vi "Update Default Template from Metadata.vi"(8 "error in":errorcluster, 9 "project refnum":refnum<vi>, 10 "measurement_signature":T2, 11 "gRPCid in":T1) -> (0 "error out":errorcluster, 1 "default value":variant, 2 "copy template path":path, 3 "gRPCid out":T1)   [LabVIEW 2021, in "MeasurementClient Editor.lvlib"]
uses:
  MeasurementClient Editor.lvlib
  <vilib>/gRPC/Generated APIs/ni/measurementlink/measurement/v2/Measurement Service Client V2/RPC Messages/ni_measurementlink_measurement_v2_MeasurementSignature.ctl
  <vilib>/gRPC/Generated APIs/ni/measurementlink/measurement/v2/Measurement Service Client V2/RPC Messages/ni_measurementlink_measurement_v2_ConfigurationParameter.ctl
  <vilib>/gRPC/Generated APIs/ni/measurementlink/measurement/v2/Measurement Service Client V2/RPC Messages/google_protobuf_Field_Kind.ctl
  <vilib>/gRPC/Generated APIs/ni/measurementlink/measurement/v2/Measurement Service Client V2/RPC Messages/ni_measurementlink_measurement_v2_ConfigurationParameter_AnnotationsEntry.ctl
  <vilib>/gRPC/Generated APIs/ni/measurementlink/measurement/v2/Measurement Service Client V2/RPC Messages/google_protobuf_Any.ctl
  <vilib>/gRPC/Generated APIs/ni/measurementlink/measurement/v2/Measurement Service Client V2/RPC Messages/ni_measurementlink_measurement_v2_Output.ctl
  <vilib>/gRPC/Generated APIs/ni/measurementlink/measurement/v2/Measurement Service Client V2/RPC Messages/ni_measurementlink_measurement_v2_Output_AnnotationsEntry.ctl
  <vilib>/gRPC/LabVIEW gRPC Library/Shared/grpcId.ctl
  <vilib>/Utility/traverseref.llb/TRef TravTarget.ctl
  <vilib>/gRPC/LabVIEW gRPC Library/grpc-lvsupport-release.lvlib
  <vilib>/Utility/traverseref.llb/VI Scripting - Traverse.lvlib
  <vilib>/gRPC/Generated APIs/ni/measurementlink/measurement/v2/Measurement Service Client V2/Measurement Service Client V2.lvlib
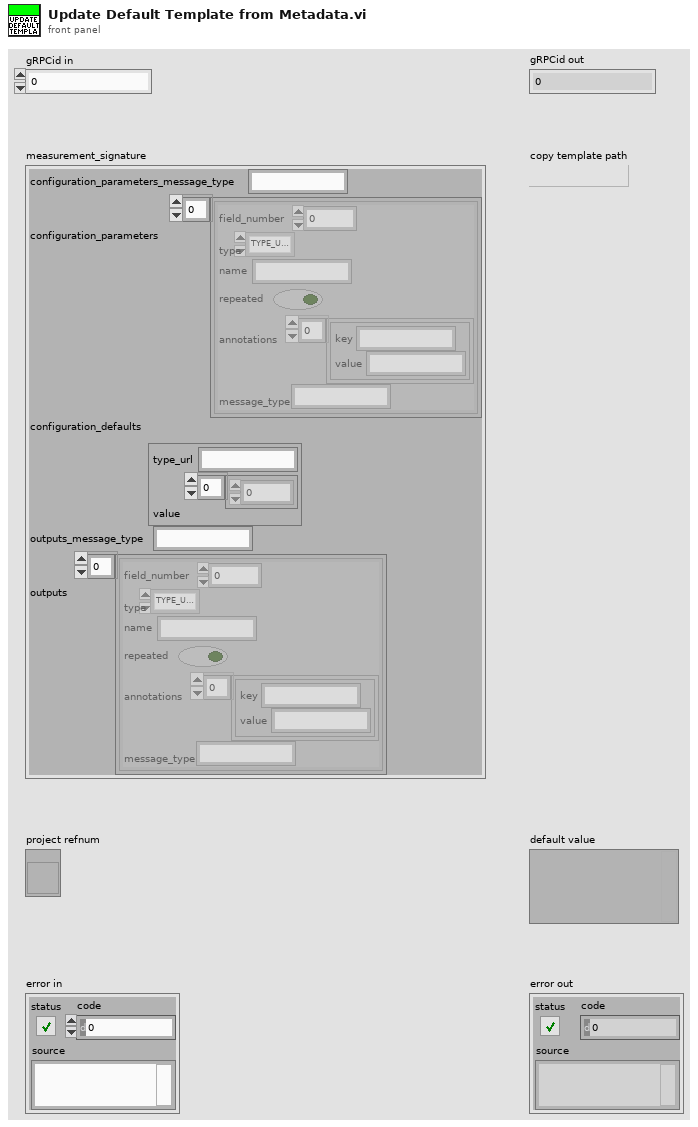
[diagram p1: front panel]
types:
  T1 = typedef "grpc-lvsupport-release.lvlib/grpcId.ctl" = u64
  T2 = typedef "Measurement Service Client V2.lvlib/ni_measurementlink_measurement_v2_MeasurementSignature.ctl" = cluster{"configuration_parameters_message_type":string, "configuration_parameters":T3[], "configuration_defaults":T6, "outputs_message_type":string, "outputs":T7[]}
  T3 = typedef "Measurement Service Client V2.lvlib/ni_measurementlink_measurement_v2_ConfigurationParameter.ctl" = cluster{"field_number":i32, "type":T4, "name":string, "repeated":bool, "annotations":T5[], "message_type":string}
  T4 = typedef "Measurement Service Client V2.lvlib/google_protobuf_Field_Kind.ctl" = enum32{"TYPE_UNKNOWN", "TYPE_DOUBLE", "TYPE_FLOAT", "TYPE_INT64", "TYPE_UINT64", "TYPE_INT32", "TYPE_FIXED64", "TYPE_FIXED32", "TYPE_BOOL", "TYPE_STRING", "TYPE_GROUP", "TYPE_MESSAGE", "TYPE_BYTES", "TYPE_UINT32", "TYPE_ENUM", "TYPE_SFIXED32", "TYPE_SFIXED64", "TYPE_SINT32", "TYPE_SINT64"}
  T5 = typedef "Measurement Service Client V2.lvlib/ni_measurementlink_measurement_v2_ConfigurationParameter_AnnotationsEntry.ctl" = cluster{"key":string, "value":string}
  T6 = typedef "Measurement Service Client V2.lvlib/google_protobuf_Any.ctl" = cluster{"type_url":string, "value":u8[]}
  T7 = typedef "Measurement Service Client V2.lvlib/ni_measurementlink_measurement_v2_Output.ctl" = cluster{"field_number":i32, "type":T4, "name":string, "repeated":bool, "annotations":T8[], "message_type":string}
  T8 = typedef "Measurement Service Client V2.lvlib/ni_measurementlink_measurement_v2_Output_AnnotationsEntry.ctl" = cluster{"key":string, "value":string}
  T9 = typedef "TRef TravTarget.ctl" = enum16{"FP", "BD", "Other"}
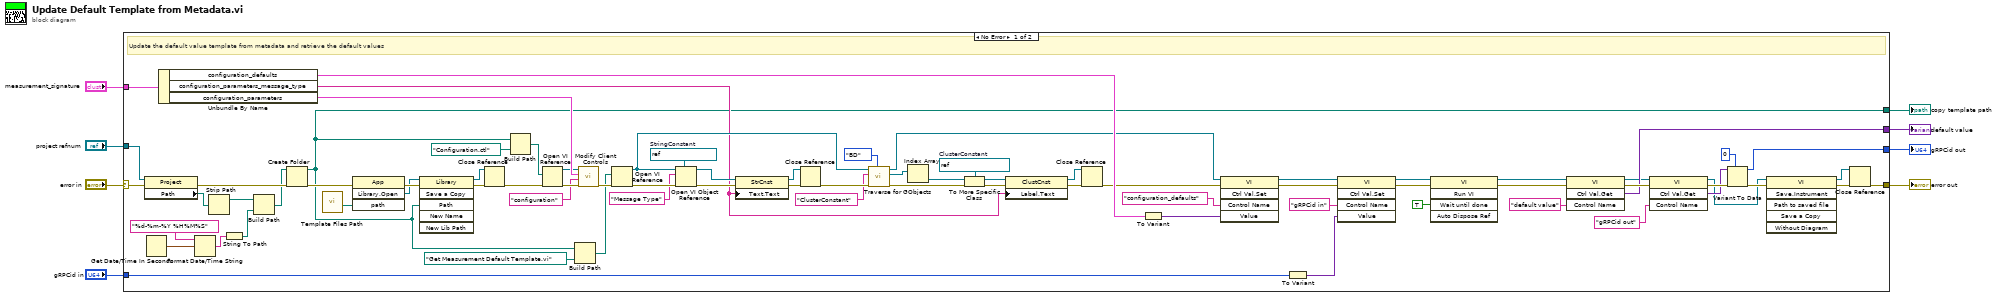
[diagram p0: block diagram]
diagram:
  n1 = case shown="No Error" "error in" {
    selector: "error in" -> [w85 w87]
    tunnel: [w73 w87] -> w7
    tunnel: "measurement_signature" -> [w67 _]
    tunnel: "gRPCid in" -> [w64 w86]
    tunnel: [w55 _] -> w3
    tunnel: [w47 w86] -> w4
    tunnel: "project refnum" -> [w32 _]
    tunnel: [w10 _] -> w1
    frame No Error {
      w38 = refnum<vi> refnum  # ClusterConstant
      w79 = refnum<vi> refnum  # StringConstant
      # "Update the default value template from metadata and retrieve the default values"
      n2 = property class="Project"(reference=w32, error in=w85) -> (error out=w28:errorcluster, "Path"=w31:path)  [unwired: 1 out]
      n3 = Get Date/Time In Seconds() -> (seconds since 1Jan1904=w30:timestamp)
      n4 = Unbundle By Name(w67) -> ("configuration_defaults"=w69:T6, "configuration_parameters_message_type"=w35:string, "configuration_parameters"=w84:T3[])
      n5 = Format Date/Time String(time format string (%c)="%d-%m-%Y %H%M%S", seconds (now)=w30) -> (date/time string=w19:string)  [unwired: 1 in]
      n6 = Strip Path(path=w31) -> (stripped path=w29:path)  [unwired: 1 out]
      n7 = String To Path(string=w19) -> (path=w20:path)
      n8 = Build Path(base path=w29, name or relative path=w20) -> (appended path=w26:path)
      n9 = Create Folder(path (use dialog)=w26, error in=w28) -> (created path=w10:path, error out=w27:errorcluster)  [unwired: 1 in, 1 out]
      n10 = call "Template Files Path.vi"() -> ("default template path"=w9:path)  [unwired: 9 in, 2 out]
      n11 = invoke class="App" method="Library.Open"(error in=w27, "path"=w9) -> (error out=w16:errorcluster, "Open Library"=w14:refnum<vi>)  [unwired: 2 in, 2 out]
      n12 = invoke class="Library" method="Save a Copy"(reference=w14, error in=w16, "Path"=w10) -> (reference out=w11:refnum<vi>, error out=w15:errorcluster)  [unwired: 3 in, 4 out]
      n13 = Close Reference(reference=w11, error in (no error)=w15) -> (error out=w12:errorcluster)
      n14 = Build Path(base path=w10, name or relative path=path "Configuration.ctl") -> (appended path=w24:path)
      n15 = Open VI Reference(vi path=w24, error in (no error)=w12) -> (vi reference=w23:refnum<vi>, error out=w25:errorcluster)  [unwired: 4 in]
      n16 = Build Path(base path=w10, name or relative path=path "Get Measurement Default Template.vi") -> (appended path=w21:path)
      n17 = call "Modify Client Controls.vi"("error in"=w25, "control name"="configuration", "parameter data"=w84, "vi refnum"=w23) -> ("error out"=w83:errorcluster)  [unwired: 7 in]
      n18 = Open VI Reference(vi path=w21, error in (no error)=w83) -> (vi reference=w42:refnum<vi>, error out=w82:errorcluster)  [unwired: 4 in]
      n19 = Open VI Object Reference(7:w79, 8:w82, 10:"Message Type" ("name/order"), 11:w42) -> (0:w80:errorcluster, 3:w77:refnum<vi>)
      n20 = property class="StrCnst"(reference=w77, error in=w80, "Text.Text"=w35) -> (reference out=w76:refnum<vi>, error out=w78:errorcluster)
      n21 = Close Reference(reference=w76, error in (no error)=w78) -> (error out=w75:errorcluster)
      n22 = call <vilib>:"Traverse for GObjects.vi"("Traverse Target"=TRef_TravTarget."BD", "error in (no error)"=w75, "Class Name"="ClusterConstant", "VI Refnum"=w42) -> ("error out"=w39:errorcluster, "References"=w43:refnum<vi>[], "dup VI Refnum"=w46:refnum<vi>)  [unwired: 4 in, 1 out]
      n23 = Index Array(array=w43) -> (element=w37:refnum<vi>)  [unwired: 1 in]
      n24 = To More Specific Class(target class=w38, reference=w37, error in=w39) -> (specific class reference=w36:refnum<vi>, error out=w40:errorcluster)
      n25 = property class="ClustCnst"(reference=w36, error in=w40, "Label.Text"=w35) -> (reference out=w33:refnum<vi>, error out=w41:errorcluster)
      n26 = Close Reference(reference=w33, error in (no error)=w41) -> (error out=w34:errorcluster)
      n27 = To Variant(anything=w69) -> (Variant=w68:variant)
      n28 = invoke class="VI" method="Ctrl Val.Set"(reference=w46, error in=w34, "Control Name"="configuration_defaults", "Value"=w68) -> (reference out=w65:refnum<vi>, error out=w71:errorcluster)  [unwired: 1 in, 3 out]
      n29 = To Variant(anything=w64) -> (Variant=w63:variant)
      n30 = invoke class="VI" method="Ctrl Val.Set"(reference=w65, error in=w71, "Control Name"="gRPCid in", "Value"=w63) -> (reference out=w60:refnum<vi>, error out=w66:errorcluster)  [unwired: 1 in, 3 out]
      n31 = invoke class="VI" method="Run VI"(reference=w60, error in=w66, "Wait until done"=TRUE ("Wait Until Done")) -> (reference out=w57:refnum<vi>, error out=w61:errorcluster)  [unwired: 2 in, 3 out]
      n32 = invoke class="VI" method="Ctrl Val.Get"(reference=w57, error in=w61, "Control Name"="default value") -> (reference out=w53:refnum<vi>, error out=w58:errorcluster, "Get Control Value Variant"=w55:variant)  [unwired: 1 in, 1 out]
      n33 = invoke class="VI" method="Ctrl Val.Get"(reference=w53, error in=w58, "Control Name"="gRPCid out") -> (reference out=w49:refnum<vi>, error out=w54:errorcluster, "Get Control Value Variant"=w50:variant)  [unwired: 1 in, 1 out]
      n34 = Variant To Data(error in=w54, type=T1 0 ("gRPCid in"), Variant=w50) -> (data=w47:T1, error out=w51:errorcluster)
      n35 = invoke class="VI" method="Save.Instrument"(reference=w49, error in=w51) -> (reference out=w72:refnum<vi>, error out=w74:errorcluster)  [unwired: 4 in, 4 out]
      n36 = Close Reference(reference=w72, error in (no error)=w74) -> (error out=w73:errorcluster)
    }
    frame Error {
      # "Pass"
    }
  }
  "error out" <- w7
  "gRPCid out" <- w4
  "default value" <- w3
  "copy template path" <- w1
